vi "unit_to_multiplicator.vi"(1 "time unit":enum16{"s", "ms", "us", "ns"}(ring)) -> (0 "multiplicator":dbl)   [LabVIEW 2011]
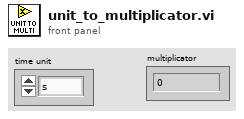
[diagram p1: front panel]
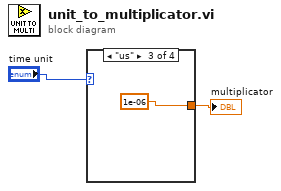
[diagram p0: block diagram]
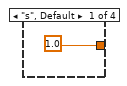
[diagram p2: hidden frame]
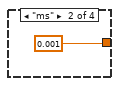
[diagram p3: hidden frame]
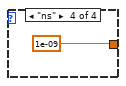
[diagram p4: hidden frame]
diagram:
  n1 = case shown="\"us\"" "time unit" {
    tunnel: [1.0 0.001 1e-06 1e-09] -> w2
    frame "s", Default {
    }
    frame "ms" {
    }
    frame "us" {
    }
    frame "ns" {
    }
  }
  "multiplicator" <- w2
